vi "Wait for Condition.vi"(8 "error in (no error)":errorcluster, 9 "FPGA Refnum in":T1, 10 "Condition checking interval":u32=50, 11 "Message Data":variant) -> (0 "error out":errorcluster, 3 "Timeout?":bool)   [LabVIEW 2018]
doc: "Waits for a certain condition to occur on either the temperature, pH, or digital trigger inputs. The condition is defined as either greater than, less than, or equal to a user specified value. If this condition does not occur before the prescribed timeout, the VI returns with the Timeout? flag set to True."
uses:
  controls/FPGA VI Reference.ctl
  controls/Condition Cluster.ctl
  <vilib>/Utility/error.llb/Error Cluster From Error Code.vi
  <vilib>/rvi/errors/niLvFpgaAdjustHostInterfaceError.vi
  <vilib>/rvi/interface/nirviReadWriteControl/nirviReadWriteControl.xnode
  NiFpgaLv.dll
  <vilib>/rvi/interface/Simulation/niFpgaSimulationCallBeginRW.vi
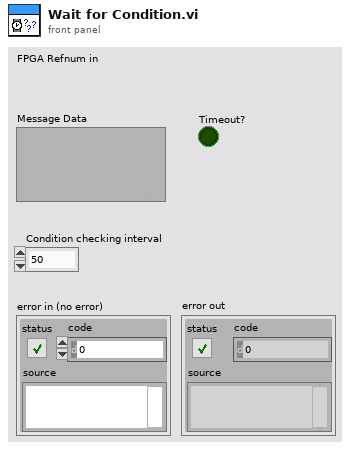
[diagram p1: front panel]
types:
  T1 = typedef "FPGA VI Reference.ctl" = refnum<k20>
  T2 = typedef "Condition Cluster.ctl" = cluster{"Condition":enum16{"Temperature", "pH", "Digital Trigger"}, "Comparison":enum16{"Greater Than", "Less Than", "Equal"}, "Condition Value":dbl, "Timeout":dbl}
  T3 = cluster{"Channel 0":fxp<+/-,20,5>, "Channel 1":fxp<+/-,20,5>, "Channel 2":bool}
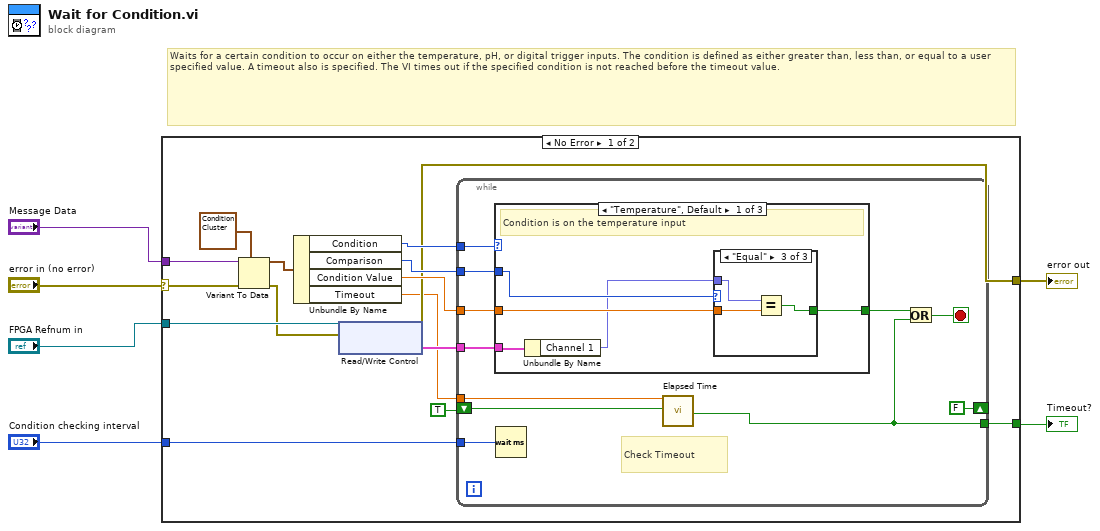
[diagram p0: block diagram]
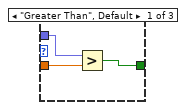
[diagram p2: hidden frame]
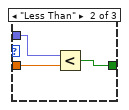
[diagram p3: hidden frame]
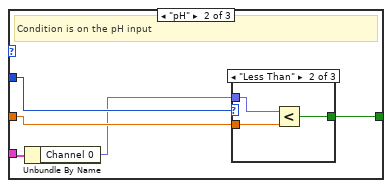
[diagram p4: hidden frame]
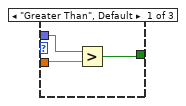
[diagram p5: hidden frame]
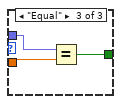
[diagram p6: hidden frame]
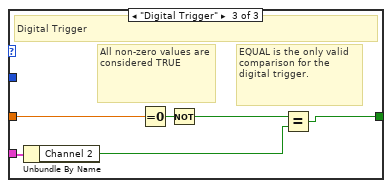
[diagram p7: hidden frame]
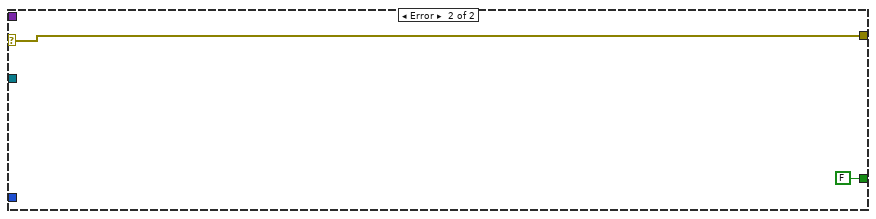
[diagram p8: hidden frame]
diagram:
  # "Waits for a certain condition to occur on either the temperature, pH, or digital trigger inputs. The condition is defined as either greater than, less than, or equal to a user specified value. A timeout also is specified. The VI times out if the specified condition is not reached before the timeout value."
  n1 = case shown="No Error" "error in (no error)" {
    selector: "error in (no error)" -> [w14 w68]
    tunnel: "FPGA Refnum in" -> [w13 _]
    tunnel: "Message Data" -> [w16 _]
    tunnel: "Condition checking interval" -> [w15 _]
    tunnel: [w10 w68] -> w3
    tunnel: [w7 FALSE ("Time has Elapsed")] -> w1
    frame No Error {
      n2 = Variant To Data(error in=w14, type=T2 {"Condition"=enum."Temperature", "Comparison"=enum."Greater Than", "Condition Value"=0.0, "Timeout"=0.0}, Variant=w16) -> (data=w18:T2, error out=w12:errorcluster)
      n3 = Unbundle By Name(w18) -> ("Condition"=w19:enum16{"Temperature", "pH", "Digital Trigger"}, "Comparison"=w20:enum16{"Greater Than", "Less Than", "Equal"}, "Condition Value"=w21:dbl, "Timeout"=w9:dbl)
      n4 = xnode "Read/Write Control"("FPGA VI Reference In"=w13, "error in"=w12) -> ("error out"=w10:errorcluster, "Input Values"=w11:T3)  [unwired: 1 out]
      n5 = while {
        tunnel: w19 -> [w32]
        tunnel: w20 -> [w31]
        tunnel: w21 -> [w30]
        tunnel: w15 -> [w29]
        tunnel: w11 -> [w28]
        tunnel: w9 -> [w27]
        shift-right: [FALSE] -> _
        shift-left: TRUE -> [w26]
        tunnel: [w22] -> w7
        stop <- w23 stop-if-true
        # "Check Timeout"
        n6 = case shown="\"Temperature\", Default" w32 {
          tunnel: w31 -> [w37 w50 _]
          tunnel: w30 -> [w36 w51 w66]
          tunnel: [w35 w49 w64] -> w24
          tunnel: w28 -> [w34 w48 w63]
          frame "Temperature", Default {
            # "Condition is on the temperature input"
            n7 = Unbundle By Name(w34) -> ("Channel 1"=w33:fxp<+/-,20,5>)
            n8 = case shown="\"Equal\"" w37 {
              tunnel: w36 -> [w40 w43 w45]
              tunnel: [w39 w42 w46] -> w35
              tunnel: w33 -> [w38 w41 w44]
              frame "Greater Than", Default {
                n9 = Greater?(x=w38, y=w40) -> (0:w39:bool)
              }
              frame "Less Than" {
                n10 = Less?(x=w41, y=w43) -> (x < y?=w42:bool)
              }
              frame "Equal" {
                n11 = Equal?(x=w44, y=w45) -> (x = y?=w46:bool)
              }
            }
          }
          frame "pH" {
            # "Condition is on the pH input"
            n12 = Unbundle By Name(w48) -> ("Channel 0"=w47:fxp<+/-,20,5>)
            n13 = case shown="\"Less Than\"" w50 {
              tunnel: w51 -> [w54 w57 w59]
              tunnel: [w53 w56 w60] -> w49
              tunnel: w47 -> [w52 w55 w58]
              frame "Greater Than", Default {
                n14 = Greater?(x=w52, y=w54) -> (0:w53:bool)
              }
              frame "Less Than" {
                n15 = Less?(x=w55, y=w57) -> (x < y?=w56:bool)
              }
              frame "Equal" {
                n16 = Equal?(x=w58, y=w59) -> (x = y?=w60:bool)
              }
            }
          }
          frame "Digital Trigger" {
            # "EQUAL is the only valid comparison for the digital trigger."
            # "All non-zero values are considered TRUE"
            # "Digital Trigger"
            n17 = Unbundle By Name(w63) -> ("Channel 2"=w62:bool)
            n18 = Equal To 0?(x=w66) -> (x = 0?=w65:bool)
            n19 = Not(x=w65) -> (.not. x?=w61:bool)
            n20 = Equal?(x=w61, y=w62) -> (x = y?=w64:bool)
          }
        }
        n21 = Wait (ms)(milliseconds to wait=w29) -> ()  [unwired: 1 out]
        n22 = call "Elapsed Time"("Time Target (s)"=w27, "Reset"=w26) -> ("Time has Elapsed"=w22:bool)  [unwired: 10 in, 7 out]
        n23 = Or(x=w24, y=w22) -> (x .or. y?=w23:bool)
      }
    }
    frame Error {
    }
  }
  "error out" <- w3
  "Timeout?" <- w1
